vi "insert.vi"(5 "replace entry if exists (F)":bool, 6 "call chain index (1)":i32=1, 7 "vi ref (caller)":refnum<vi>, 8 "error in (no error)":errorcluster, 11 "controls plan":string) -> (0 "error out":errorcluster)   [LabVIEW 2024, in "controls manager.lvlib"]
uses:
  controls manager.lvlib
  insert or remove.ctl
  entry type.ctl
  control.ctl
  controls plan.ctl
  key value pair.ctl
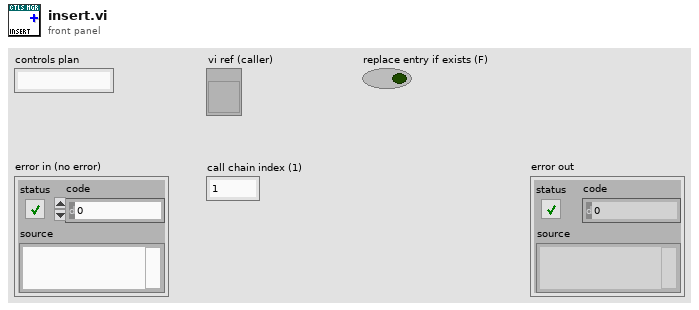
[diagram p1: front panel]
types:
  T1 = typedef "controls manager.lvlib/control.ctl" = cluster{"refnum":refnum<vi>, "index":i32}
  T2 = typedef "controls manager.lvlib/entry type.ctl" = cluster{"controls":map{string, T1}, "plan":T3}
  T3 = typedef "controls manager.lvlib/controls plan.ctl" = map{string, T4[]}
  T4 = typedef "controls manager.lvlib/key value pair.ctl" = cluster{"key":string, "value":string}
  T5 = typedef "controls manager.lvlib/insert or remove.ctl" = enum16{"insert", "remove"}
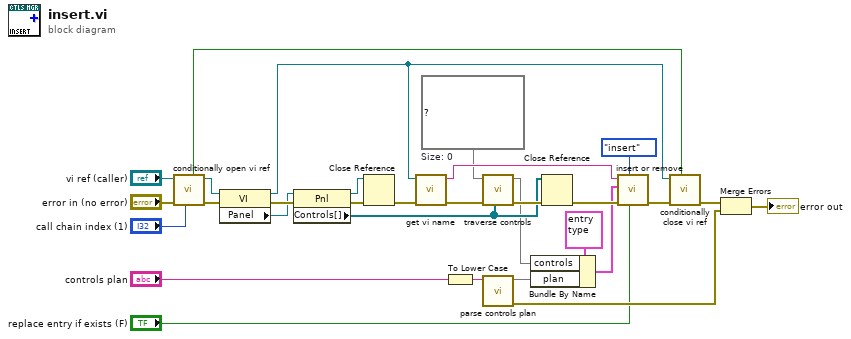
[diagram p0: block diagram]
diagram:
  w1 = map{string, T1} {}  # Size: 0
  n1 = call "conditionally open vi ref.vi"("call chain index (1)"="call chain index (1)", "error in (no error)"="error in (no error)", "vi ref in"="vi ref (caller)") -> ("error out"=w24:errorcluster, "vi ref out"=w14:refnum<vi>, "new ref?"=w18:bool)  [unwired: 6 in]
  n2 = property class="VI"(reference=w14, error in=w24) -> (reference out=w13:refnum<vi>, error out=w15:errorcluster, "Panel"=w11:refnum<vi>)
  n3 = property class="Pnl"(reference=w11, error in=w15) -> (reference out=w9:refnum<vi>, error out=w12:errorcluster, "Controls[]"=w28:refnum<vi>[])
  n4 = Close Reference(reference=w9, error in (no error)=w12) -> (error out=w10:errorcluster)
  n5 = call "get vi name.vi"("error in (no error)"=w10, "vi ref"=w13) -> ("error out"=w22:errorcluster, "vi name"=w23:string)  [unwired: 8 in]
  n6 = To Lower Case(string="controls plan") -> (all lower case string=w3:string)
  n7 = call "traverse controls.vi"("controls"=w28, "error in (no error)"=w22, "controls map in"=w1) -> ("error out"=w29:errorcluster, "controls map out"=w2:map{string, T1})  [unwired: 7 in]
  n8 = call "parse controls plan.vi"("plan in"=w3) -> ("error out"=w27:errorcluster, "plan out"=w7:T3)  [unwired: 9 in]
  n9 = Bundle By Name(cluster=T2 {"controls"={}, "plan"={}}, "controls"=w2, "plan"=w7) -> (w5:T2)
  n10 = Close Reference(reference=w28, error in (no error)=w29) -> (error out=w30:errorcluster)
  n11 = call "insert or remove.vi"("replace entry if exists"="replace entry if exists (F)", "action"=insert_or_remove."insert", "error in (no error)"=w30, "entry"=w5, "id"=w23) -> ("error out"=w21:errorcluster)  [unwired: 6 in]
  n12 = call "conditionally close vi ref.vi"("new ref?"=w18, "error in (no error)"=w21, "vi ref"=w13) -> ("error out"=w19:errorcluster)  [unwired: 8 in]
  n13 = Merge Errors(w19, w27) -> (→"error out":errorcluster)
